vi "gfitsio-get-column-info.vi"(6 "row (-1: don't check descriptor)":i32=-1, 7 "column":string, 8 "error in (no error)":errorcluster, 9 "case sensitive? (F:No)":bool, 11 "gfits refnum":T2) -> (0 "error out":errorcluster, 1 "variable length array?":bool, 2 "nelements":i32, 3 "dup gfits refnum":T2, 4 "column number":i32, 5 "cfitsio datatype":T1=1 items=["TBIT"=1, "TBYTE  (U8)"=11, "TSBYTE  (I8)"=12, "TLOGICAL"=14, "TSTRING"=16, "TUSHORT  (U16)"=20, "TSHORT  (I16)"=21, "TUINT"=31, "TULONG  (U32)"=40, "TLONG  (I32)"=41, "TFLOAT  (SGL)"=42, "TLONGLONG  (I64)"=81, "TDOUBLE  (DBL)"=82, "TCOMPLEX  (CSG)"=83, "TDOUBLECOMPLEX  (CDB)"=163])   [LabVIEW 2024, in "gfitsio.lvlib"]
doc: "Return the data type of a column in an ASCII or binary table. In the case of scaled integer columns it returns the 'equivalent' data type that is needed to store the scaled values, and not necessarily the physical data type of the unscaled values as stored in the FITS table. For example if a '1I' column in a binary table has TSCALn = 1 and TZEROn = 32768, then this column effectively contains unsigned short integer values, and thus the returned value of typecode will be TUSHORT, not TSHORT. Similarly, if a column has TTYPEn = '1I' and TSCALn = 0.12, then the returned typecode will be TFLOAT."
uses:
  gfitsio.lvlib
  gfitsio-refnum.ctl
  cfitsio-datatypes.ctl
  gfitsio.dll
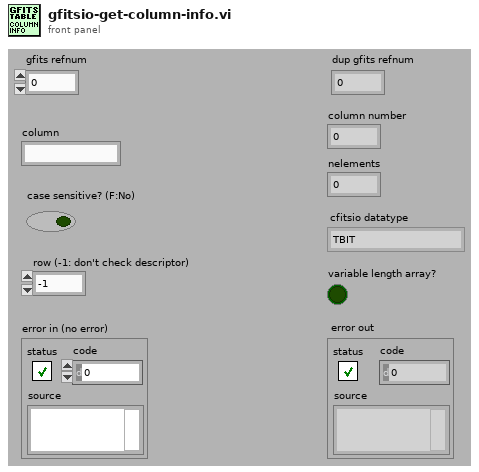
[diagram p1: front panel]
types:
  T1 = typedef "gfitsio.lvlib/cfitsio-datatypes.ctl" = i32
  T2 = typedef "gfitsio.lvlib/gfitsio-refnum.ctl" = u64
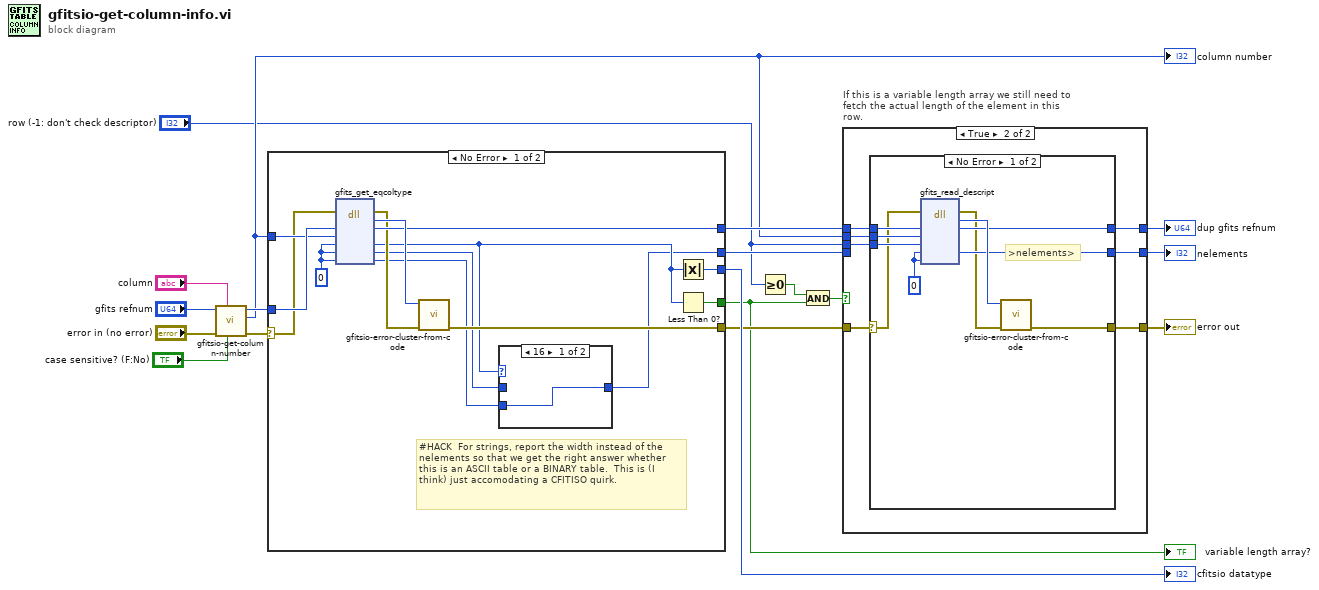
[diagram p0: block diagram]
diagram:
  n1 = call "gfitsio-get-column-number.vi"("case sensitive? (F:No)"="case sensitive? (F:No)", "column"="column", "error in (no error)"="error in (no error)", "gfits refnum"="gfits refnum") -> ("error out"=w15:errorcluster, "colnum"=w8:i32, "dup gfits refnum"=w13:T2)  [unwired: 5 in]
  "column number" <- w8
  n2 = case shown="No Error" w15 {
    selector: w15 -> [w25 w36]
    tunnel: [w31 w36] -> w11
    tunnel: w13 -> [w29 w35]
    tunnel: [w30 w35] -> w10
    tunnel: w8 -> [w28 _]
    tunnel: [w27 _] -> w18
    tunnel: [w26 _] -> w2
    tunnel: [w19 _] -> w6
    frame No Error {
      w23 = 0
      # "#HACK  For strings, report the width instead of the nelements so that we get the right answer whether this is an ASCII table or a BINARY table.  This is (I think) just accomodating a CFITISO quirk."
      n3 = dll-call lib="C:/Users/smaher/Downloads/gfitsio_v5.2_Apr_2014/gfitsio/gfitsio.dll" fn="gfits_get_eqcoltype"(error in=w25, "refnum"=w29, "colnum"=w28, "datatype"=w23, "nelements"=w23, "width"=w23) -> (error out=w24:errorcluster, "return type"=w32:i32, "refnum"=w30:T2, "datatype"=w22:i32, "nelements"=w20:i32, "width"=w21:i32)  [unwired: 3 in, 1 out]
      n4 = call "gfitsio-error-cluster-from-code.vi"("error in (no error)"=w24, "error code"=w32) -> ("error out"=w31:errorcluster)  [unwired: 9 in]
      n5 = case shown="16" w22 {
        tunnel: w20 -> [_ w34]
        tunnel: w21 -> [w33 _]
        tunnel: [w33 w34] -> w19
        frame 16 {
        }
        frame Default {
        }
      }
      n6 = Absolute Value(x=w22) -> (abs(x)=w27:i32)
      n7 = Less Than 0?(x=w22) -> (x < 0?=w26:bool)
    }
    frame Error {
    }
  }
  "cfitsio datatype" <- w18
  "variable length array?" <- w2
  n8 = Greater Or Equal To 0?(x="row (-1: don't check descriptor)") -> (x >= 0?=w4:bool)
  n9 = And(x=w4, y=w2) -> (x .and. y?=w3:bool)
  n10 = case "If this is a variable length array we still need to fetch the actual length of the element in this row." shown="True" w3 {
    tunnel: [w37 w46] -> w1
    tunnel: [w38 w45] -> w9
    tunnel: [w39 w44] -> w7
    tunnel: "row (-1: don't check descriptor)" -> [_ w43]
    tunnel: w11 -> [w37 w42]
    tunnel: w10 -> [w38 w41]
    tunnel: w8 -> [_ w40]
    tunnel: w6 -> [w39 _]
    frame False {
      # ">nelements>"
    }
    frame True {
      n11 = case shown="No Error" w42 {
        selector: w42 -> [w48 w58]
        tunnel: [w55 w58] -> w46
        tunnel: w41 -> [w53 w57]
        tunnel: [w54 w57] -> w45
        tunnel: [w49 _] -> w44
        tunnel: w40 -> [w52 _]
        tunnel: w43 -> [w50 _]
        frame No Error {
          w51 = 0
          # ">nelements>"
          n12 = dll-call lib="C:/Users/smaher/Downloads/gfitsio_v5.2_Apr_2014/gfitsio/gfitsio.dll" fn="gfits_read_descript"(error in=w48, "refnum"=w53, "colnum"=w52, "row"=w50, "nelements"=w51, "offset"=w51) -> (error out=w47:errorcluster, "return type"=w56:i32, "refnum"=w54:T2, "nelements"=w49:i32)  [unwired: 4 in, 2 out]
          n13 = call "gfitsio-error-cluster-from-code.vi"("error in (no error)"=w47, "error code"=w56) -> ("error out"=w55:errorcluster)  [unwired: 9 out]
        }
        frame Error {
        }
      }
    }
  }
  "error out" <- w1
  "dup gfits refnum" <- w9
  "nelements" <- w7
